vi "setAxisTitle.vi"(8 "Error In":errorcluster, 9 "title":string, 10 "axisId":T1 items=["yLeft", "yRight", "xBottom", "xTop"], 11 "LQChart In":refnum<class "LQChart.lvclass">) -> (0 "Error Out":errorcluster, 3 "LQChart Out":refnum<class "LQChart.lvclass">)   [LabVIEW 2014, in "LQChart.lvclass"]
doc: "LabVIEW-specific documentation is not yet available."
uses:
  LQChart.lvclass
  Qwt/QwtPlot/Axis.ctl
  LQ Core/LQIdentity/LQIdentity.lvclass/LQIdentity.ctl
  LQ Core/LQ Core.lvlib
  LQ Core/LQIdentity/LQIdentity.lvclass
  Qwt/QwtPlot/QwtPlot.lvclass
panel:
  # "Copyright (c) 2016 Sze Howe Koh\n\nThis Source Code Form is subject to the terms of the Mozilla Public\nLicense, v. 2.0. If a copy of the MPL was not distributed with this\nfile, You can obtain one at http://mozilla.org/MPL/2.0/."
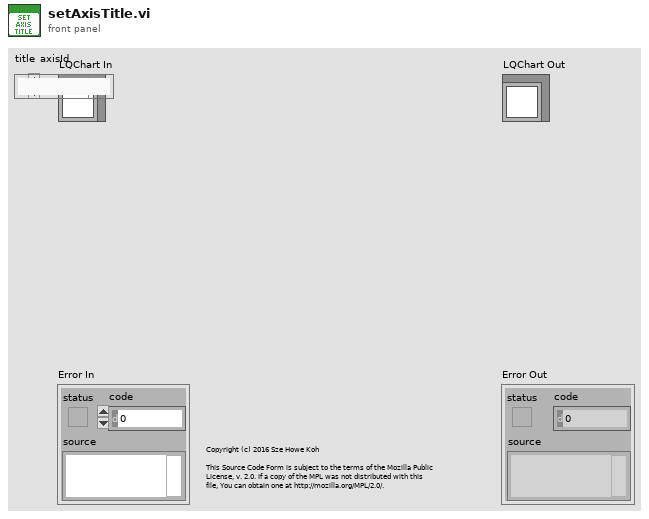
[diagram p1: front panel]
types:
  T1 = typedef "QwtPlot.lvclass/Axis.ctl" = i32
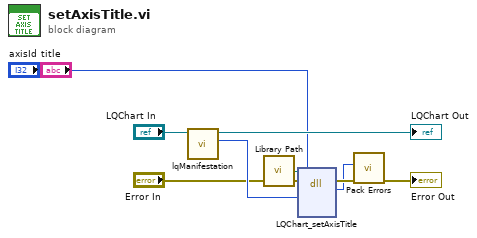
[diagram p0: block diagram]
diagram:
  n1 = call "lqManifestation.vi"("LQIdentity in"="LQChart In") -> ("Manifestation"=w7:u64, "LQIdentity out"=→"LQChart Out":refnum<class "LQChart.lvclass">)  [unwired: 9 in]
  n2 = call "Library Path.vi"() -> ("Library Path"=w8:path)
  n3 = dll-call lib="?" fn="LQChart_setAxisTitle"(path in=w8, error in="Error In", "_instance"=w7, "axisId"="axisId", "title"="title") -> (error out=w5:errorcluster, w3:i32)  [unwired: 4 in, 1 out]
  n4 = call "Pack Errors.vi"("Error In"=w5, "Error Code"=w3) -> ("Error Out"=→"Error Out":errorcluster)  [unwired: 9 in]
